vi "Generate Unique Name.vi"(8 "error in (no error)":errorcluster, 10 "Type":string, 11 "Da Base in":refnum<class "Template Module.lvclass">) -> (0 "error out":errorcluster, 2 "Unique name":string, 3 "Da Base out":refnum<class "Template Module.lvclass">)   [LabVIEW 2019, in "Template Module.lvclass"]
uses:
  Template Module.lvclass
  Template Module.lvclass/Template Module.ctl
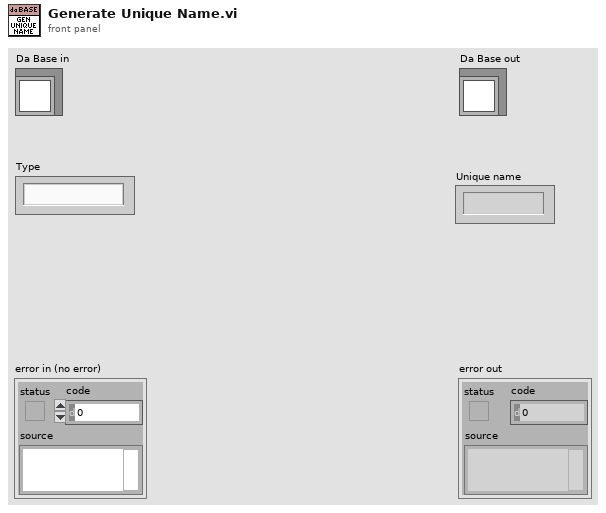
[diagram p1: front panel]
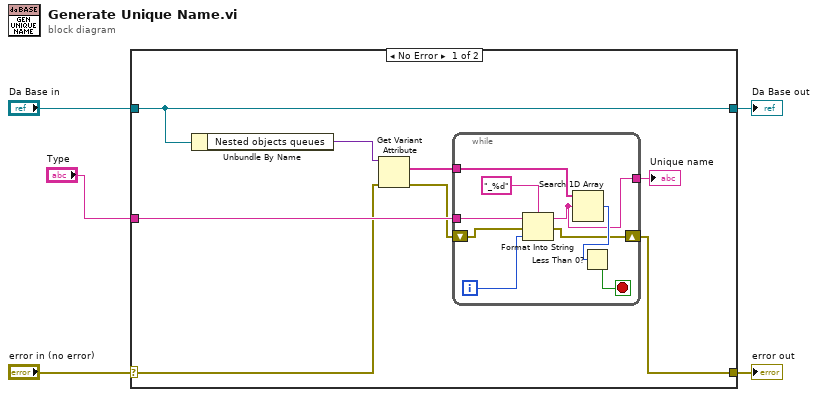
[diagram p0: block diagram]
diagram:
  n1 = case shown="No Error" "error in (no error)" {
    selector: "error in (no error)" -> [w7 w24]
    tunnel: [w6 w24] -> w4
    tunnel: [w13 w23] -> w2
    tunnel: "Da Base in" -> [w13 w23]
    tunnel: "Type" -> [w10 _]
    frame No Error {
      n2 = Unbundle By Name(w13) -> ("Nested objects queues"=w12:variant)
      n3 = Get Variant Attribute(Variant=w12, error in=w7) -> (names=w11:string[], error out=w9:errorcluster)  [unwired: 2 in, 2 out]
      n4 = while {
        tunnel: w11 -> [w18]
        tunnel: w10 -> [w21]
        shift-right: [w15] -> w6
        shift-left: w9 -> [w19]
        tunnel: [w14] -> w8
        i -> [w22]
        stop <- w16 stop-if-true
        n5 = Format Into String(format string="_%d", initial string=w21, error in=w19, w22) -> (resulting string=w14:string, error out=w15:errorcluster)
        n6 = Search 1D Array(1D array=w18, element=w14) -> (index of element=w17:i32)  [unwired: 1 in]
        n7 = Less Than 0?(x=w17) -> (x < 0?=w16:bool)
      }
      "Unique name" <- w8
    }
    frame Error {
    }
  }
  "error out" <- w4
  "Da Base out" <- w2
